vi "Write Player Info.vi"(8 "error in (no error)":errorcluster, 10 "Player Info":T1={"Name"="Spread", "Color Box"=0, "Gloat Phrase"="Let Chaos Rule"}, 11 "Attack in":refnum<class "Spread.lvclass">) -> (0 "error out":errorcluster, 3 "Attack out":refnum<class "Spread.lvclass">)   [LabVIEW 2014, in "Spread.lvclass"]
uses:
  Spread.lvclass
  Player Info.ctl
  Square.lvclass
  SquareBattle Arena/SquareBattle Arena.lvclass
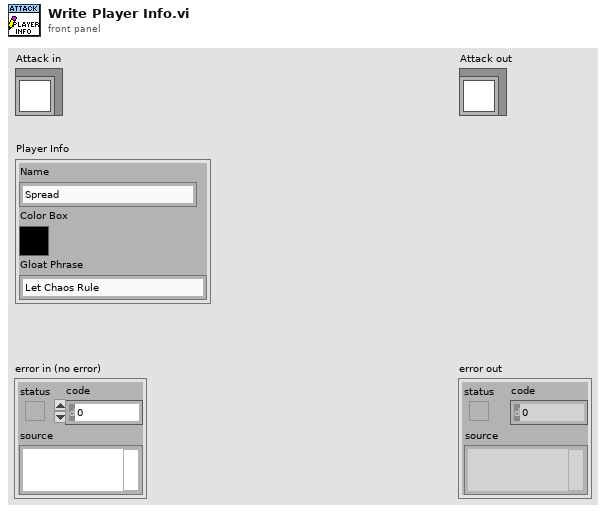
[diagram p1: front panel]
types:
  T1 = typedef "SquareBattle Arena.lvlib/SquareBattle Arena.lvclass/Player Info.ctl" = cluster{"Name":string, "Color Box":u32, "Gloat Phrase":string}
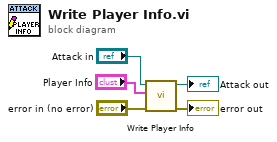
[diagram p0: block diagram]
diagram:
  n1 = call-parent "Write Player Info.vi"("error in (no error)"="error in (no error)", "Player Info"="Player Info", "Runner in"="Attack in") -> ("error out"=→"error out":errorcluster, "Runner out"=→"Attack out":refnum<class "Spread.lvclass">)  [unwired: 7 in]
